vi "Estimate All Positions.vi"(0 "Position Estimation Method":u32(ring) items=["Star Configuration", "Swarm Method"]) -> ()   [LabVIEW 2014, in "Position.lvclass"]
doc: "Choose a method for position estimation."
uses:
  Position.lvclass
  Tag.lvclass
  Anchor/Anchor.lvclass
panel:
  in  "Enable Error margin?":bool
  in  "DistanceLimitTag":dbl=70.0
  in  "Error Margin":dbl=2.0
  out "error out":errorcluster
  in  "error in (no error)":errorcluster
  out "Output AnchorArray":refnum<class "Anchor.lvclass">[](array[class])
  out "Intersections":T1(array[cluster])
  out "PositionCluster [tagID, x, y, anchorID, distances]":T2
  in  "Input AnchorArray":refnum<class "Anchor.lvclass">[](array[class])
  in  "TagDistanceArray":T3(array[cluster])
  in  "Tag.lvclass":refnum<class "Tag.lvclass">
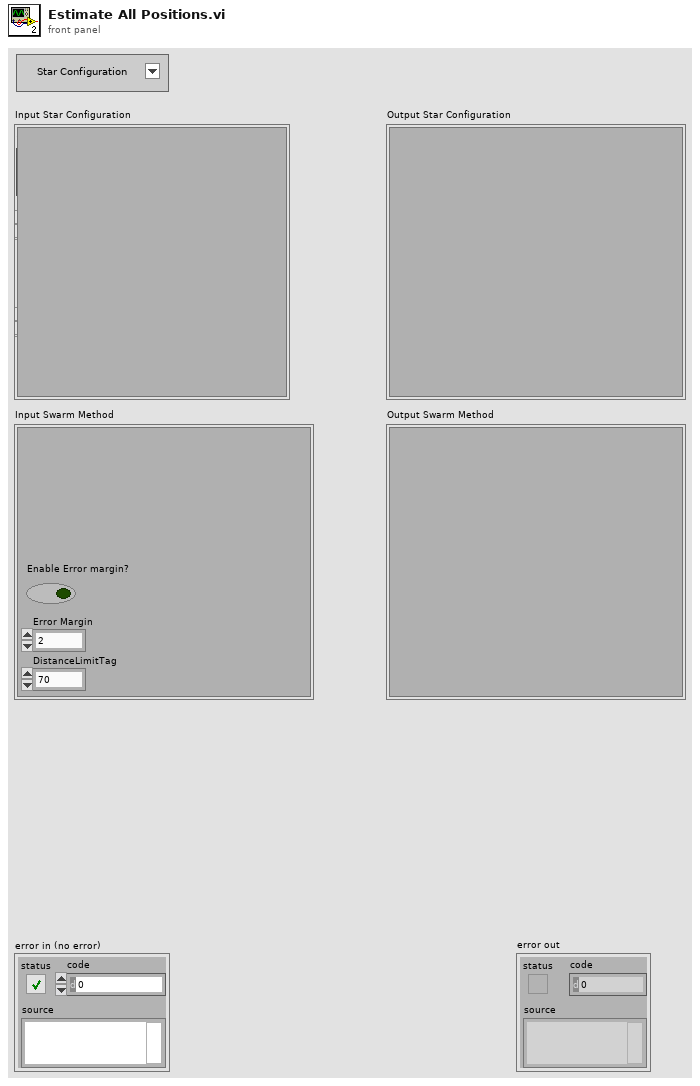
[diagram p1: front panel]
types:
  T1 = cluster{"time [ms]":dbl, "x":dbl, "y":dbl, "Fout":bool, "Goed":bool}[]
  T2 = cluster{"tagID":dbl, "X":dbl, "Y":dbl, "anchorIDDistanceCluster":cluster{"anchorIDArray":dbl[], "anchorDistanceArray":dbl[]}}
  T3 = cluster{"TagDistance":dbl, "Tag To":refnum<class "Tag.lvclass">, "Tag From":refnum<class "Tag.lvclass">}[]
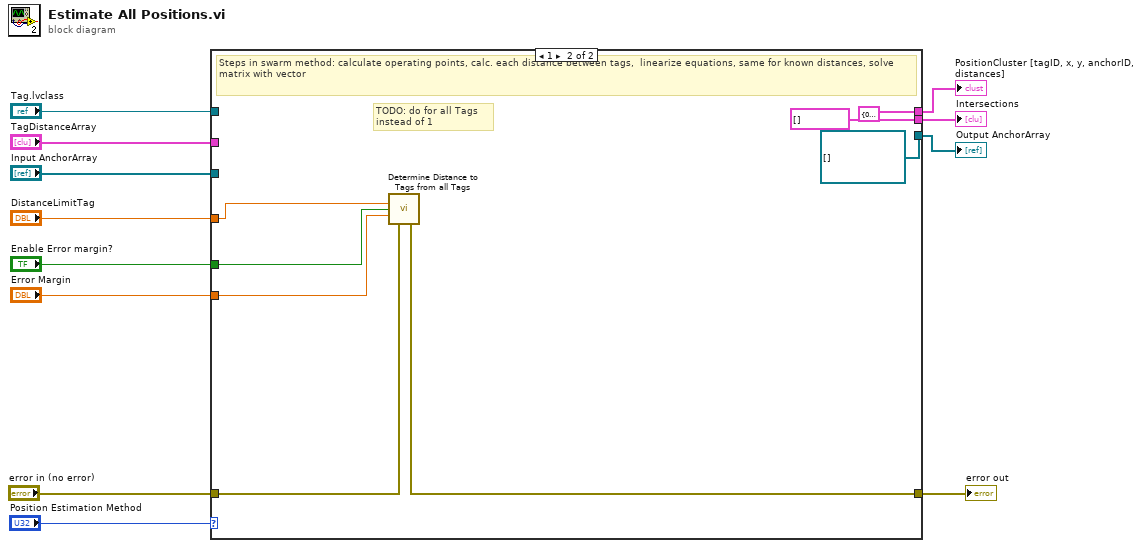
[diagram p0: block diagram]
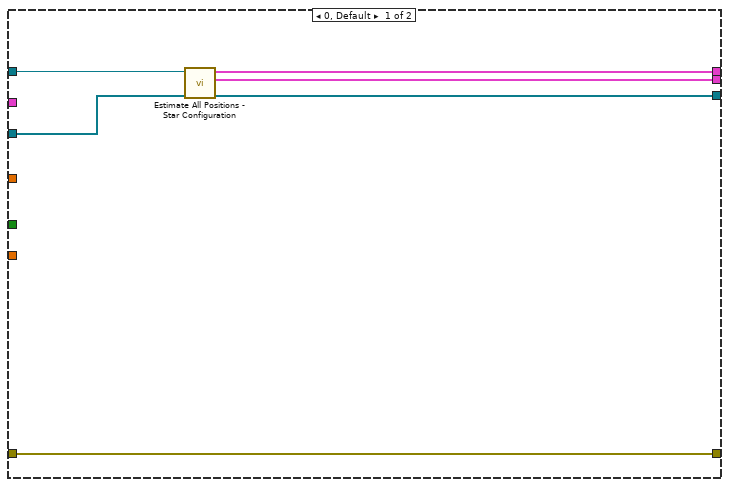
[diagram p2: hidden frame]
diagram:
  n1 = case shown="1" "Position Estimation Method" {
    tunnel: "Tag.lvclass" -> [w18 _]
    tunnel: "TagDistanceArray" -> [_ _]
    tunnel: "Input AnchorArray" -> [w17 _]
    tunnel: [w16 refnum<class "Anchor.lvclass">[] [] ("Output AnchorArray")] -> w6
    tunnel: [w15 T1 [] ("Intersections")] -> w7
    tunnel: [w14 T2 {"tagID"=0.0, "X"=0.0, "Y"=0.0, "anchorIDDistanceCluster"={"anchorIDArray"=[], "anchorDistanceArray"=[]}} ("PositionCluster [tagID, x, y, anchorID, distances]")] -> w8
    tunnel: "error in (no error)" -> [w13 w23]
    tunnel: [w13 w22] -> w4
    tunnel: "Error Margin" -> [_ w24]
    tunnel: "DistanceLimitTag" -> [_ w20]
    tunnel: "Enable Error margin?" -> [_ w21]
    frame 0, Default {
      n2 = call "Estimate All Positions - Star Configuration.vi"("Input AnchorArray"=w17, "Tag.lvclass"=w18) -> ("Output AnchorArray"=w16:refnum<class "Anchor.lvclass">[], "Intersections"=w15:T1, "PositionCluster [tagID, x, y, anchorID, distances]"=w14:T2)  [unwired: 7 in]
    }
    frame 1 {
      # "TODO: do for all Tags\ninstead of 1"
      # "Steps in swarm method: calculate operating points, calc. each distance between tags,  linearize equations, same for known distances, solve matrix with vector"
      n3 = call "Determine Distance to Tags from all Tags.vi"("DistanceLimitTag"=w20, "Enable Error margin?"=w21, "Error Margin"=w24, "error in (no error)"=w23) -> ("error out"=w22:errorcluster)  [unwired: 10 in, 1 out]
    }
  }
  "PositionCluster [tagID, x, y, anchorID, distances]" <- w8
  "Intersections" <- w7
  "Output AnchorArray" <- w6
  "error out" <- w4
